vi "Create Linear Waveform File.vi"(6 "error in":errorcluster, 9 "filename":path=path "C:/ATS Development/Code/Test Cases/Tools/Waveform DC 0 volts.dat") -> (0 "error out":errorcluster, 3 "Waveform":waveform(dbl)(graph))   [LabVIEW 2010]
uses:
  <vilib>/Waveform/WDTFileIO.llb/ Write Waveform to File.vi
panel:
  in  "append file (F)":bool
  in  "nelem (1000)":i32=1000
  in  "start (0.0)":dbl format="%.3f"
  in  "step (0.0)":dbl format="%.3f"
  in  "parameters":waveform(dbl)={"t0"=timestamp(3473168073.631 s since 1904-01-01), "dt"=0.001, "Y"=[], "attributes"=variant("Average Size"=variant(dbl 15.0), "NSamp"=variant(dbl 400000.0), "Resistance (ohms)"=variant(dbl 500.0), "Samp Freq (MHz)"=variant(dbl 100.0), "dt (us)"=variant(dbl 0.01))}
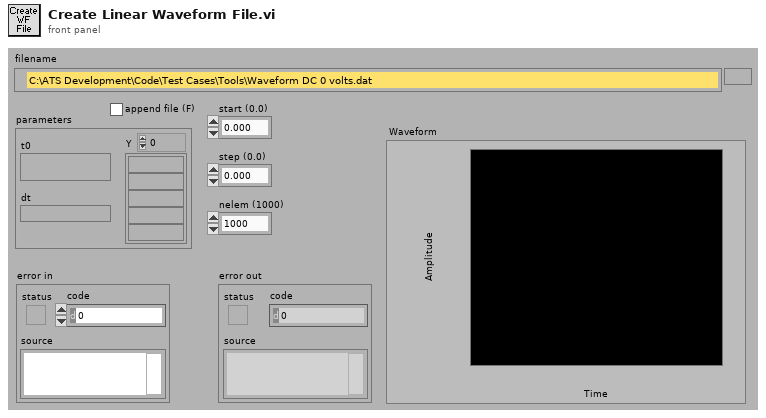
[diagram p1: front panel]
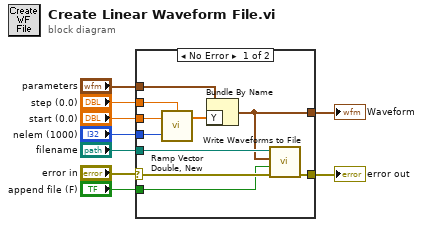
[diagram p0: block diagram]
diagram:
  n1 = case shown="No Error" "error in" {
    selector: "error in" -> [w18 w20]
    tunnel: [w19 w20] -> w8
    tunnel: "parameters" -> [w16 _]
    tunnel: "step (0.0)" -> [w15 _]
    tunnel: "start (0.0)" -> [w14 _]
    tunnel: "nelem (1000)" -> [w13 _]
    tunnel: "filename" -> [w12 _]
    tunnel: [w11 _] -> w2
    tunnel: "append file (F)" -> [w10 _]
    frame No Error {
      n2 = call "Ramp Vector Double, New.vi"("step (1.0)"=w15, "nelem"=w13, "start (0.0)"=w14) -> ("ramp"=w17:dbl[])
      n3 = Bundle By Name(cluster=w16, "Y"=w17) -> (w11:waveform(dbl))
      n4 = call-poly <vilib>:"Write Waveforms to File.vi"("error in (no error)"=w18, "append to file? (new file:F)"=w10, "waveform"=w11, "file path (dialog if empty)"=w12) -> ("error out"=w19:errorcluster)  [unwired: 6 in, 1 out]
    }
    frame Error {
    }
  }
  "error out" <- w8
  "Waveform" <- w2
